vi "XIPIN_Floating-point_5_0.vi"   [LabVIEW 2017]
doc: "The Xilinx Floating-Point Operator is capable of being configured to provide a range of floating-point operations. The core offers addition, subtraction, multiplication, division, square-root, compare and conversion operations. High-speed, with single-cycle throughput is provided at a wide range of wordlengths that includes both single and double precision. Embedded multipliers or XtremeDSP slices can be used with certain operations.\n------------------------------------\n<b>Need License</b> : No"
uses:
  <vilib>/rvi/XilinxIP/XIPIN_XNode/niFpgaXIPIN.xnode
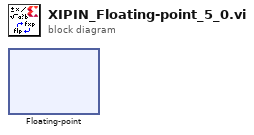
[diagram p0: block diagram]
diagram:
  n1 = xnode ("Floating-point")() -> ()
